vi "get children.vi"(8 "error in":errorcluster, 10 "ID":string, 11 "memory hierarchy":T1) -> (0 "error out":errorcluster, 1 "children":refnum<class "NISE_CEF_serializable configuration.lvclass">[](array[class]))   [LabVIEW 2013, in "NISE_CEF_TreeSerializer.lvlib"]
uses:
  NISE_CEF_TreeSerializer.lvlib
  memory hierarchy.ctl
  hierarchy element.ctl
  serializable configuration/NISE_CEF_serializable configuration.lvclass
  serializable configuration/NISE_CEF_serializable configuration.lvclass/NISE_CEF_serializable configuration.ctl
  NISE_CEF_TreeControl.lvlib
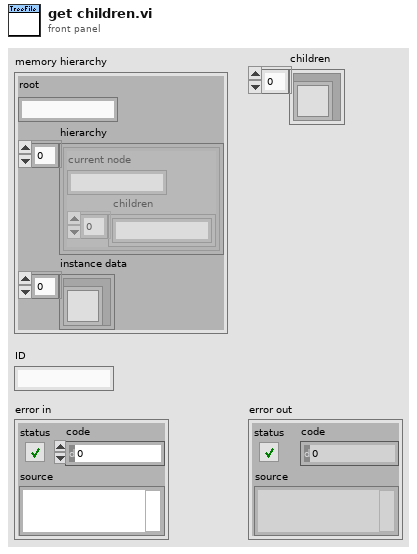
[diagram p1: front panel]
types:
  T1 = typedef "NISE_CEF_TreeSerializer.lvlib/memory hierarchy.ctl" = cluster{"root":string, "hierarchy":T2[], "instance data":refnum<class "NISE_CEF_serializable configuration.lvclass">[]}
  T2 = typedef "NISE_CEF_TreeSerializer.lvlib/hierarchy element.ctl" = cluster{"current node":string, "children":string[]}
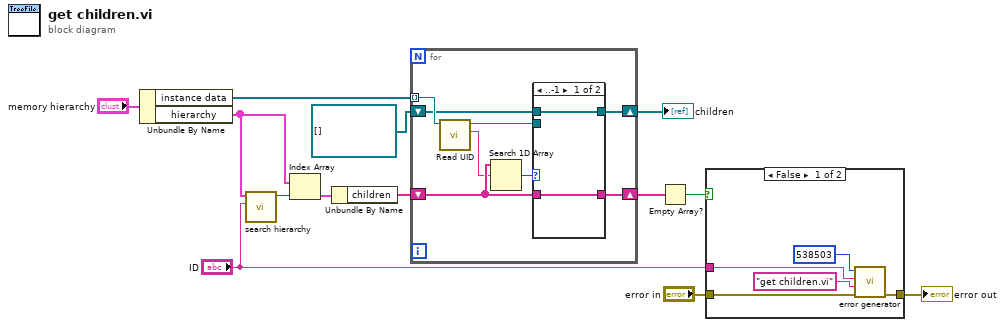
[diagram p0: block diagram]
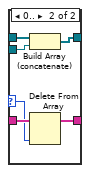
[diagram p3: hidden frame]
diagram:
  n1 = Unbundle By Name("memory hierarchy") -> ("instance data"=w9:refnum<class "NISE_CEF_serializable configuration.lvclass">[], "hierarchy"=w12:T2[])
  n2 = call "search hierarchy.vi"("ID"="ID", "hierarchy"=w12) -> ("index"=w11:i32)  [unwired: 8 in, 1 out]
  n3 = Index Array(array=w12, index=w11) -> (element=w10:T2)
  n4 = Unbundle By Name(w10) -> ("children"=w8:string[])
  n5 = for {
    tunnel: w9 -> [w21] mode=indexing
    shift-right: [w15] -> w4
    shift-left: w8 -> [w16]
    shift-right: [w18] -> w6
    shift-left: refnum<class "NISE_CEF_serializable configuration.lvclass">[] [] -> [w17]
    n6 = call "Read UID.vi"("configuration in"=w21) -> ("instance id"=w14:string, "configuration out"=w19:refnum<class "NISE_CEF_serializable configuration.lvclass">)  [unwired: 8 in, 1 out]
    n7 = Search 1D Array(1D array=w16, element=w14) -> (index of element=w20:i32)  [unwired: 1 in]
    n8 = case shown="..-1" w20 {
      selector: w20 -> [_ w25]
      tunnel: w19 -> [_ w29]
      tunnel: [w23 w28] -> w18
      tunnel: w17 -> [w23 w27]
      tunnel: w16 -> [w22 w26]
      tunnel: [w22 w24] -> w15
      frame ..-1 {
      }
      frame 0.. {
        n9 = Build Array (concatenate)(w27, w29) -> (w28:refnum<class "NISE_CEF_serializable configuration.lvclass">[])
        n10 = Delete From Array(array=w26, index=w25) -> (array with subset deleted=w24:string[])  [unwired: 1 in, 1 out]
      }
    }
  }
  "children" <- w6
  n11 = Empty Array?(array=w4) -> (empty?=w3:bool)
  n12 = case shown="False" w3 {
    tunnel: "ID" -> [w32 _]
    tunnel: "error in" -> [w31 w35]
    tunnel: [w30 w35] -> w1
    frame False {
      n13 = call "error generator.vi"("error in"=w31, "source"="get children.vi", "append error message"=w32, "error code (0)"=538503) -> ("error out"=w30:errorcluster)  [unwired: 5 in]
    }
    frame True {
    }
  }
  "error out" <- w1
